vi "Configure Chan Characteristics.vi"(0 "VISA Resource Name":refnum<visa-resource-name>, 5 "Channel Name (\"CH1\")":string(combo)="CH1", 7 "Input Impedance (1.0 mega ohm)":string(combo)="MEG", 9 "Max Input Frequency (20.0E+6 Hz)":string(combo)="TWENTY", 11 "error in (no error)":errorcluster {"code" format="%.0x"}) -> (4 "VISA Resource Name Out":refnum<visa-resource-name>, 15 "error out":errorcluster {"code" format="%.0x"})   [LabVIEW 2010, in "Tektronix TDS 3000 Series.lvlib"]
doc: "This VI configures the properties that control the electrical characteristics of the channel. These properties are the input impedance and the max input frequency."
uses:
  <instrlib>/Tektronix TDS 3000 Series/Tektronix TDS 3000 Series.lvlib
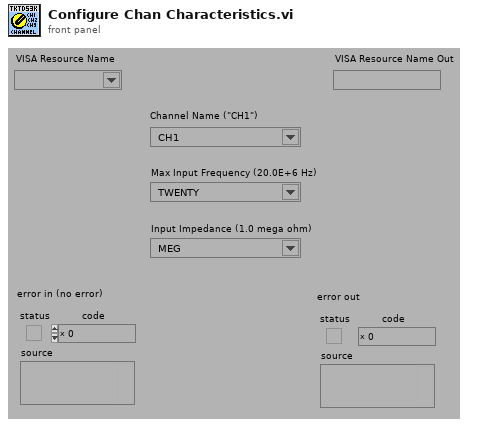
[diagram p1: front panel]
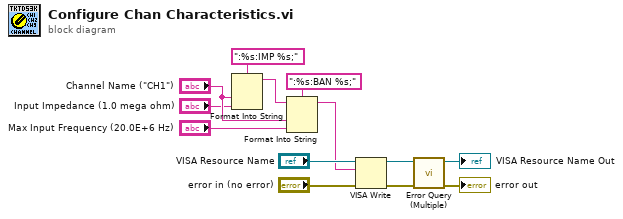
[diagram p0: block diagram]
diagram:
  n1 = Format Into String(format string=":%s:IMP %s;", "Channel Name (\"CH1\")", "Input Impedance (1.0 mega ohm)") -> (resulting string=w5:string)  [unwired: 2 in, 1 out]
  n2 = Format Into String(format string=":%s:BAN %s;", initial string=w5, "Channel Name (\"CH1\")", "Max Input Frequency (20.0E+6 Hz)") -> (resulting string=w6:string)  [unwired: 1 in, 1 out]
  n3 = VISA Write(VISA resource name="VISA Resource Name", write buffer=w6, error in (no error)="error in (no error)") -> (VISA resource name out=w4:refnum<visa-resource-name>, error out=w3:errorcluster)  [unwired: 1 out]
  n4 = call <instrlib>:"Error Query (Multiple).vi"("error in (no error)"=w3, "VISA Resource Name"=w4) -> ("error out"=→"error out":errorcluster, "VISA Resource Name Out"=→"VISA Resource Name Out":refnum<visa-resource-name>)  [unwired: 6 in, 2 out]
